vi "DataFlowTime.vi"(10 "process":string, 11 "data":T1) -> (3 "data out":T1)   [LabVIEW 2017, in "Benchmarking.lvlib"]
uses:
  <vilib>/addons/InsightCM/Devices/Shared/Common/Benchmarking/Benchmarking.lvlib
  <vilib>/addons/InsightCM/Devices/Shared/Common/DataFlow/controls/Data.ctl
  <vilib>/addons/InsightCM/Utilities/DataAccessors/controls/wfmSGL_DVR.ctl
  <vilib>/addons/PointValueMap/controls/PointMap.ctl
  <vilib>/addons/InsightCM/Devices/Shared/Common/DataFlow/controls/Type.ctl
  <vilib>/addons/PointValueMap/subVIs/Point_Read_i32.vi
  <vilib>/addons/PointValueMap/PointValueMap.lvlib
  <vilib>/addons/TraceLogger/TraceLogger.lvlib
  <vilib>/addons/InsightCM/Devices/Shared/Common/DataFlow/DataFlow.lvlib
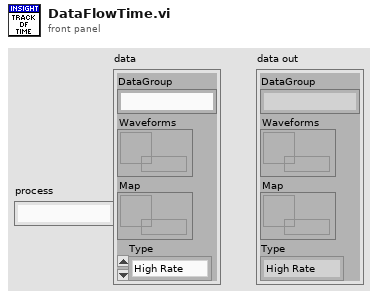
[diagram p1: front panel]
types:
  T1 = typedef "DataFlow.lvlib/Data.ctl" = cluster{"DataGroup":string, "Waveforms":T2, "Map":T3, "Type":T4}
  T2 = typedef "wfmSGL_DVR.ctl" = refnum<data-value>
  T3 = typedef "PointValueMap.lvlib/PointMap.ctl" = refnum<data-value>
  T4 = typedef "DataFlow.lvlib/Type.ctl" = enum16{"High Rate", "Low Rate", "Burst Mode"}
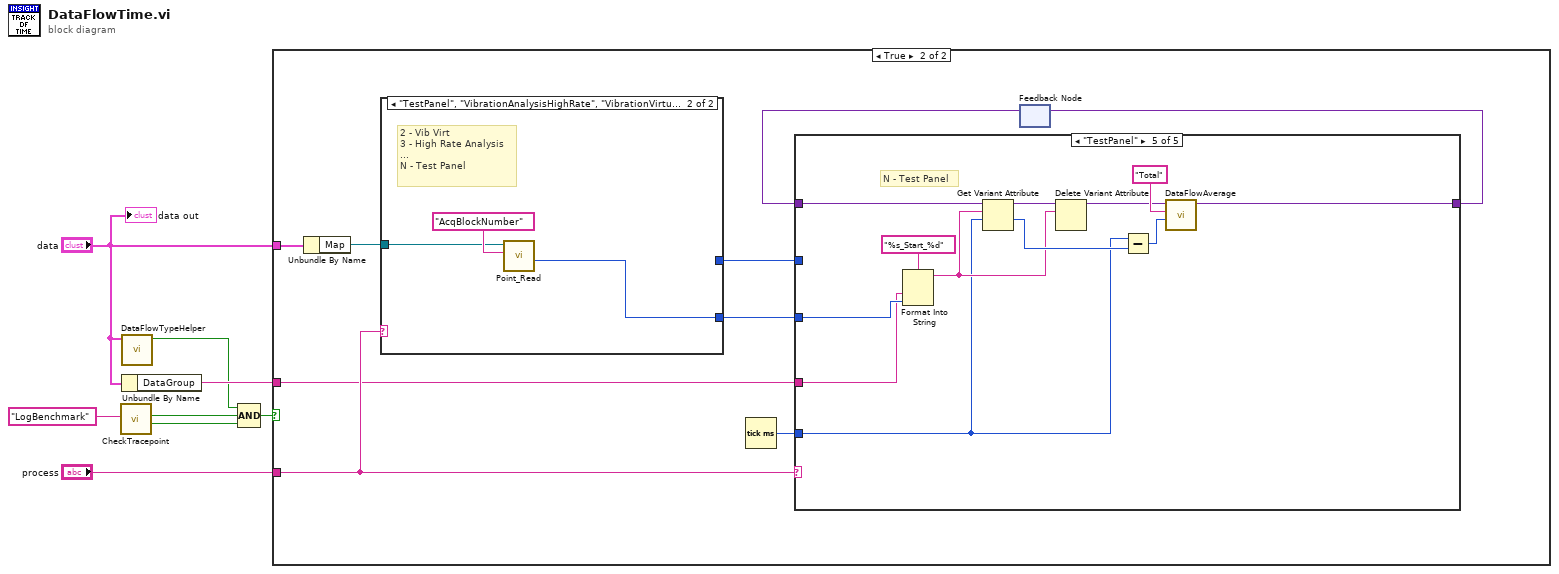
[diagram p0: block diagram]
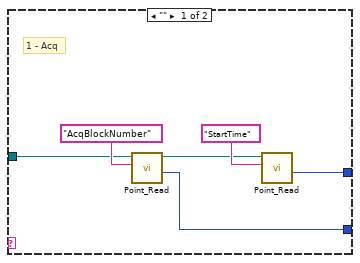
[diagram p3: hidden frame]
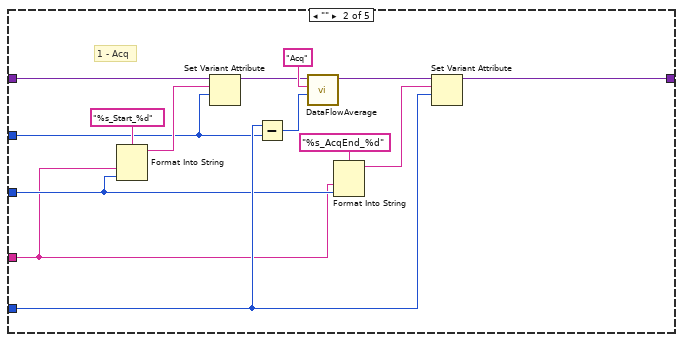
[diagram p5: hidden frame]
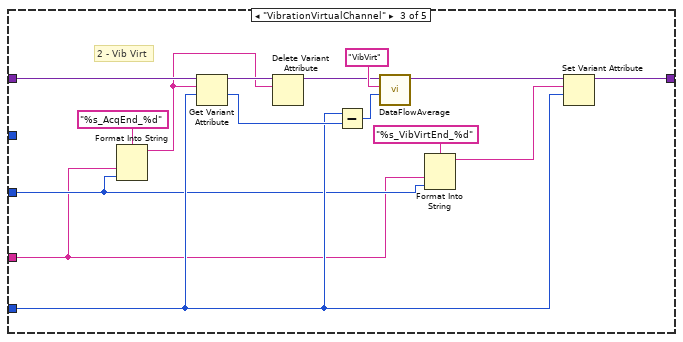
[diagram p6: hidden frame]
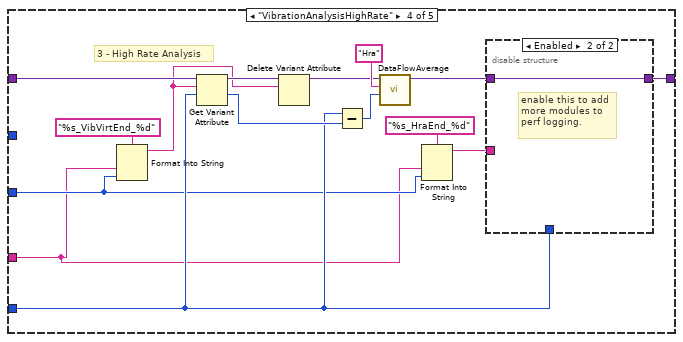
[diagram p7: hidden frame]
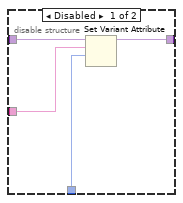
[diagram p8: hidden frame]
diagram:
  n1 = call <vilib>:"CheckTracepoint.vi"("tracepoint"="LogBenchmark") -> ("found"=w6:bool, "enabled"=w5:bool)  [unwired: 8 in, 1 out]
  n2 = call <vilib>:"DataFlowTypeHelper.vi"("data"="data") -> ("high rate"=w1:bool)  [unwired: 8 in, 2 out]
  n3 = Unbundle By Name("data") -> ("DataGroup"=w3:string)
  n4 = Compound Arithmetic op=AND(w1, w5, w6) -> (w4:bool)
  n5 = case shown="True" w4 {
    tunnel: "data" -> [_ w12]
    tunnel: "process" -> [_ w11]
    tunnel: w3 -> [_ w9]
    frame False {
    }
    frame True {
      n6 = Unbundle By Name(w12) -> ("Map"=w13:T3)
      n7 = case shown="\"TestPanel\", \"VibrationAnalysisHighRate\", \"VibrationVirtualChannel\", Default" w11 {
        tunnel: [w21 w24] -> w15
        tunnel: w13 -> [w22 w25]
        tunnel: [w18 _] -> w10
        frame "" {
          # "1 - Acq"
          n8 = call-poly <vilib>:"Point_Read.vi"("Tag"="AcqBlockNumber", "Map"=w22) -> ("Value"=w21:i32, "Map Out"=w19:T3)  [unwired: 4 in, 4 out]
          n9 = call-poly <vilib>:"Point_Read.vi"("Tag"="StartTime", "Map"=w19) -> ("Value"=w18:i32)  [unwired: 4 in, 5 out]
        }
        frame "TestPanel", "VibrationAnalysisHighRate", "VibrationVirtualChannel", Default {
          # "2 - Vib Virt\n3 - High Rate Analysis\n...\nN - Test Panel"
          n10 = call-poly <vilib>:"Point_Read.vi"("Tag"="AcqBlockNumber", "Map"=w25) -> ("Value"=w24:i32)  [unwired: 4 in, 5 out]
        }
      }
      n11 = Tick Count (ms)() -> (millisecond timer value=w14:u32)
      n12 = feedback #1() -> (w16:variant)  [unwired: 1 in]
      n13 = case shown="\"TestPanel\"" w11 {
        tunnel: [w27 w35 w50 w65 w77] -> w17
        tunnel: w16 -> [w27 w39 w53 w68 w85]
        tunnel: w15 -> [_ w29 w46 w61 w79]
        tunnel: w14 -> [_ w31 w47 w62 w80]
        tunnel: w10 -> [_ w30 _ _ _]
        tunnel: w9 -> [_ w28 w45 w60 w78]
        frame Default {
        }
        frame "" {
          # "1 - Acq"
          n14 = Format Into String(format string="%s_Start_%d", w28, w29) -> (resulting string=w37:string)  [unwired: 2 in, 1 out]
          n15 = Set Variant Attribute(Variant=w39, name=w37, value=w30) -> (Variant out=w34:variant)  [unwired: 1 in, 2 out]
          n16 = Subtract(x=w31, y=w30) -> (x-y=w40:u32)
          n17 = call <vilib>:"DataFlowAverage.vi"("timer"=w40, "name"="Acq" ("format string"), "data in"=w34) -> ("data out"=w36:variant)  [unwired: 7 in, 1 out]
          n18 = Format Into String(format string="%s_AcqEnd_%d" ("name"), w28, w29) -> (resulting string=w32:string)  [unwired: 2 in, 1 out]
          n19 = Set Variant Attribute(Variant=w36, name=w32, value=w31) -> (Variant out=w35:variant)  [unwired: 1 in, 2 out]
        }
        frame "VibrationVirtualChannel" {
          # "2 - Vib Virt"
          n20 = Format Into String(format string="%s_AcqEnd_%d", w45, w46) -> (resulting string=w42:string)  [unwired: 2 in, 1 out]
          n21 = Get Variant Attribute(Variant=w53, name=w42, default value (empty Variant)=w47) -> (duplicate Variant=w44:variant, value=w55:u32)  [unwired: 1 in, 2 out]
          n22 = Delete Variant Attribute(6:w42, 7:w44) -> (3:w43:variant)  [unwired: 1 in, 2 out]
          n23 = Subtract(x=w47, y=w55) -> (x-y=w54:u32)
          n24 = call <vilib>:"DataFlowAverage.vi"("timer"=w54, "name"="VibVirt" ("format string"), "data in"=w43) -> ("data out"=w51:variant)  [unwired: 7 in, 1 out]
          n25 = Format Into String(format string="%s_VibVirtEnd_%d" ("name"), w45, w46) -> (resulting string=w48:string)  [unwired: 2 in, 1 out]
          n26 = Set Variant Attribute(Variant=w51, name=w48, value=w47) -> (Variant out=w50:variant)  [unwired: 1 in, 2 out]
        }
        frame "VibrationAnalysisHighRate" {
          # "3 - High Rate Analysis"
          n27 = Format Into String(format string="%s_VibVirtEnd_%d", w60, w61) -> (resulting string=w57:string)  [unwired: 2 in, 1 out]
          n28 = Get Variant Attribute(Variant=w68, name=w57, default value (empty Variant)=w62) -> (duplicate Variant=w59:variant, value=w70:u32)  [unwired: 1 in, 2 out]
          n29 = Delete Variant Attribute(6:w57, 7:w59) -> (3:w58:variant)  [unwired: 1 in, 2 out]
          n30 = Subtract(x=w62, y=w70) -> (x-y=w69:u32)
          n31 = call <vilib>:"DataFlowAverage.vi"("timer"=w69, "name"="Hra" ("format string"), "data in"=w58) -> ("data out"=w66:variant)  [unwired: 7 in, 1 out]
          n32 = Format Into String(format string="%s_HraEnd_%d" ("name"), w60, w61) -> (resulting string=w63:string)  [unwired: 2 in, 1 out]
          n33 = disable-structure shown="Enabled" {
            disable-tunnel: w66 -> [w75 w76]
            disable-tunnel: [w74 w76] -> w65
            disable-tunnel: w63 -> [w73 _]
            disable-tunnel: w62 -> [w72 _]
            frame Disabled {
              n34 = Set Variant Attribute(Variant=w75, name=w73, value=w72) -> (Variant out=w74:variant)  [unwired: 1 in, 2 out]
            }
            frame Enabled {
              # "enable this to add\nmore modules to\nperf logging."
            }
          }
        }
        frame "TestPanel" {
          # "N - Test Panel"
          n35 = Format Into String(format string="%s_Start_%d", w78, w79) -> (resulting string=w81:string)  [unwired: 2 in, 1 out]
          n36 = Get Variant Attribute(Variant=w85, name=w81, default value (empty Variant)=w80) -> (duplicate Variant=w83:variant, value=w87:u32)  [unwired: 1 in, 2 out]
          n37 = Delete Variant Attribute(6:w81, 7:w83) -> (3:w82:variant)  [unwired: 1 in, 2 out]
          n38 = Subtract(x=w80, y=w87) -> (x-y=w86:u32)
          n39 = call <vilib>:"DataFlowAverage.vi"("timer"=w86, "name"="Total" ("format string"), "data in"=w82) -> ("data out"=w77:variant)  [unwired: 7 in, 1 out]
        }
      }
      n40 = feedback-in #1(w17) -> ()
    }
  }
  "data out" <- "data"
